vi "Main.vi"() -> ()   [LabVIEW 2019, in "SignalProcessor.lvlib"]
doc: "This template is based off of the Queued Message Handler design pattern and the Queued Message Handler project template that ships with LabVIEW.\n\nThe main difference is that the queue is private to this module and communication between modules is performed via Broadcast and Request events.\n\nRequest events are wrapped in public API methods and are handled in the Event Handling Loop (EHL) of this VI. Any module can register for Broadcast events sent by this module. The EHL generates messages based on user interface actions.\n\nThe Message Handling Loop (MHL) processes messages generated by the EHL, or by other messages. The messages are string values, so new messages can be added easily to the Message Cases case structure in the MHL. Each message cluster can also provide an optional value for Message Data, which is a variant that can be converted to whatever message-specific data is required.\n_____\nBased on Delacor QMH Project Template 4.2.1.64."
uses:
  SignalProcessor.lvlib
  <vilib>/Delacor/Delacor QMH/Libraries/Module Admin_class/Delacor_lib_QMH_Module Admin.lvclass
  Module Data--cluster.ctl
  <vilib>/Delacor/Delacor QMH/Libraries/Message Queue_class/Delacor_lib_QMH_Message Queue.lvclass/Delacor_lib_QMH_Message Queue.ctl
  Stop Argument--cluster.ctl
  <vilib>/Delacor/Delacor QMH/Libraries/Module Admin_class/Delacor_lib_QMH_Module Admin.lvclass/Delacor_lib_QMH_Module Admin.ctl
  ProcessWaveform Argument--cluster.ctl
  <vilib>/Utility/miscctls.llb/LVPointTypeDef.ctl
  <vilib>/Delacor/Delacor QMH/Libraries/Message Queue_class/Delacor_lib_QMH_Enqueue Message (Single).vi
  <vilib>/Delacor/Delacor QMH/Libraries/Module Admin_class/Delacor_lib_QMH_Get External Launch.vi
  <vilib>/Analysis/baseanly.llb/Mean (DBL).vi
  <vilib>/Analysis/5stat.llb/RMS (DBL).vi
  <vilib>/Utility/error.llb/Error Cluster From Error Code.vi
  <vilib>/Waveform/WDTOps.llb/WDT Waveform Duration DBL.vi
  <vilib>/ErrorRing/Error Ring.xnode
  <vilib>/Delacor/Delacor QMH/Libraries/Message Queue_class/Delacor_lib_QMH_Message Queue.lvclass
  <vilib>/Analysis/NI_AALPro.lvlib
  <vilib>/Analysis/NI_AALBase.lvlib
panel:
  in  "Simulate MHL Error":bool
  in  "Simulate EHL Error":bool
  out "error out":errorcluster
  in  "Module Admin":refnum<class "Delacor_lib_QMH_Module Admin.lvclass">
  out "Status":string
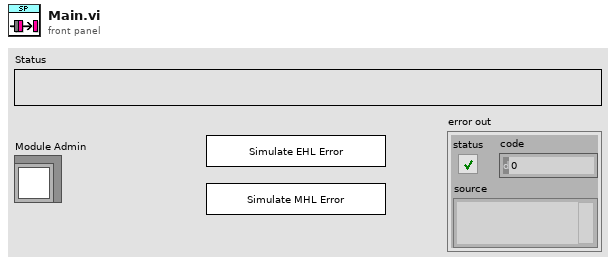
[diagram p1: front panel]
types:
  T1 = typedef "SignalProcessor.lvlib/Request Events--cluster.ctl" = cluster{"Stop Module":refnum<user-event>, "Show Panel":refnum<user-event>, "Hide Panel":refnum<user-event>, "Get Module Execution Status":refnum<user-event>, "Show Diagram":refnum<user-event>, "ProcessWaveform":refnum<user-event>}
  T2 = typedef "SignalProcessor.lvlib/Module Data--cluster.ctl" = cluster{"Status":string}
  T3 = enum32{"invalid lock state", "Not Locked", "Locked (No Password)", "Password-protected"}
  T4 = typedef "SignalProcessor.lvlib/Stop Argument--cluster.ctl" = cluster{"Origin":string, "Exit via Stop Module Req?":bool, "Wait for Module to stop?":bool}
  T5 = typedef "SignalProcessor.lvlib/ProcessWaveform Argument--cluster.ctl" = cluster{"Data":waveform(dbl)}
  T6 = typedef "LVPointTypeDef.ctl" = cluster{"Horizontal":i16, "Vertical":i16}
  T7 = enum32{"Invalid", "Standard", "Closed", "Hidden", "Minimized", "Maximized"}
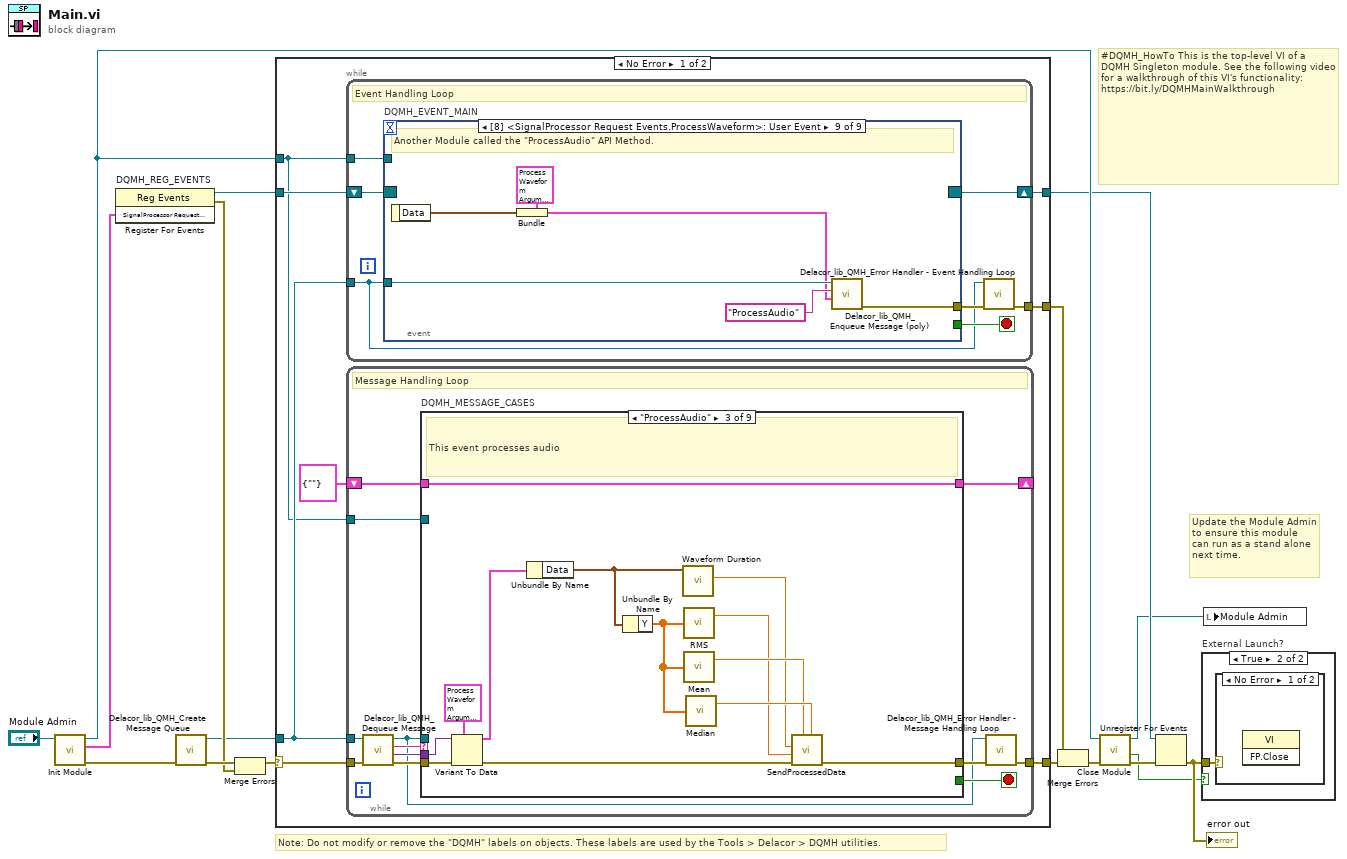
[diagram p0: block diagram]
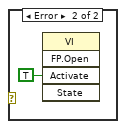
[diagram p3: hidden frame]
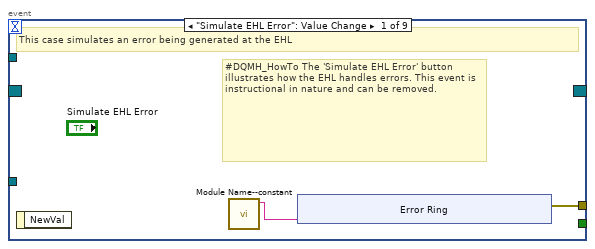
[diagram p4: hidden frame]
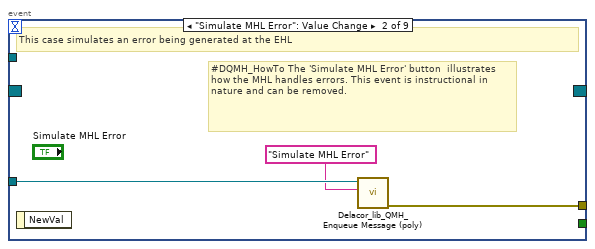
[diagram p5: hidden frame]
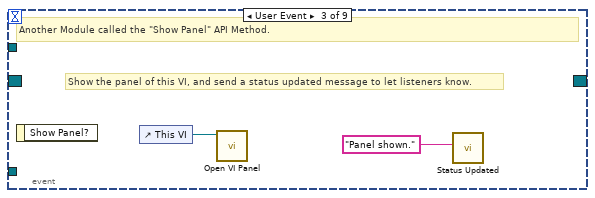
[diagram p6: hidden frame]
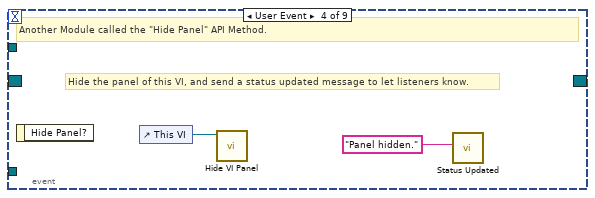
[diagram p7: hidden frame]
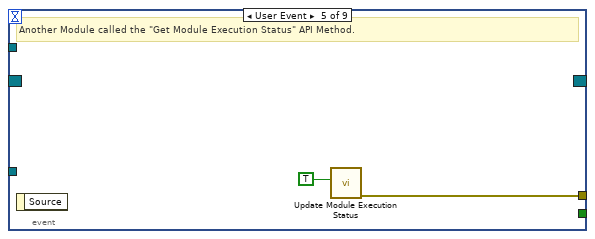
[diagram p8: hidden frame]
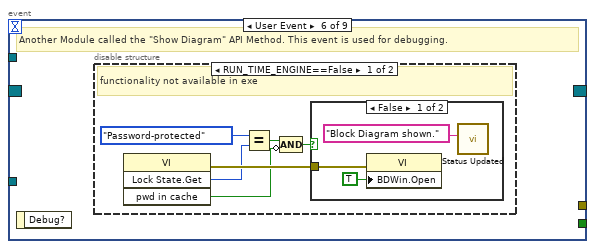
[diagram p9: hidden frame]
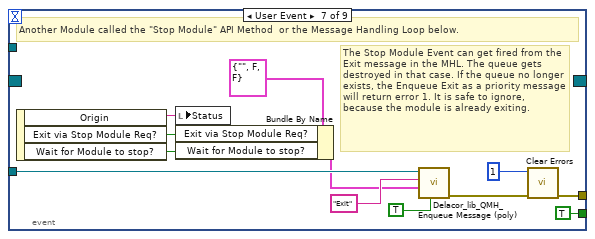
[diagram p12: hidden frame]
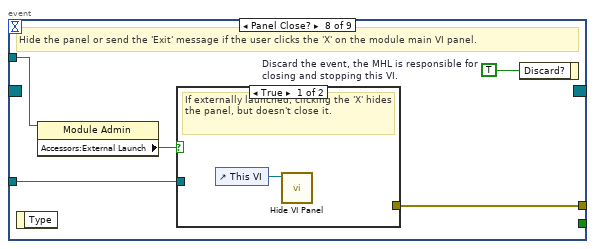
[diagram p13: hidden frame]
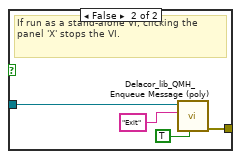
[diagram p14: hidden frame]
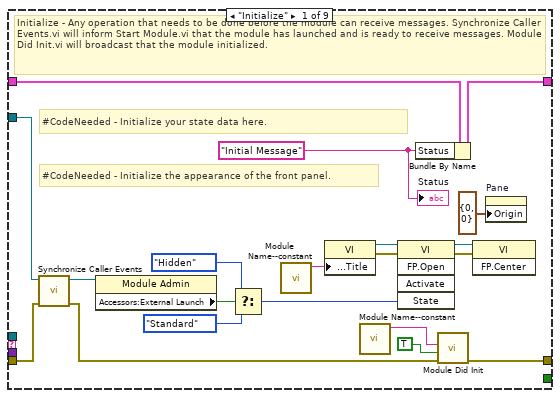
[diagram p15: hidden frame]
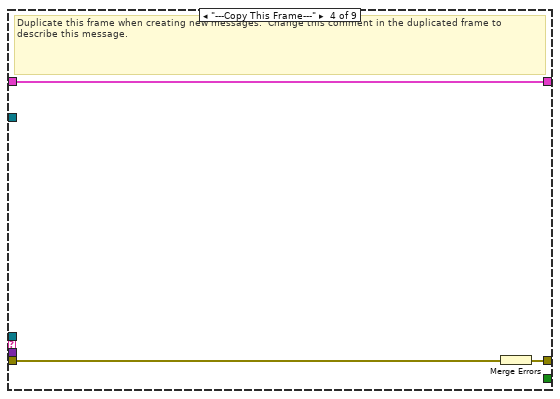
[diagram p17: hidden frame]
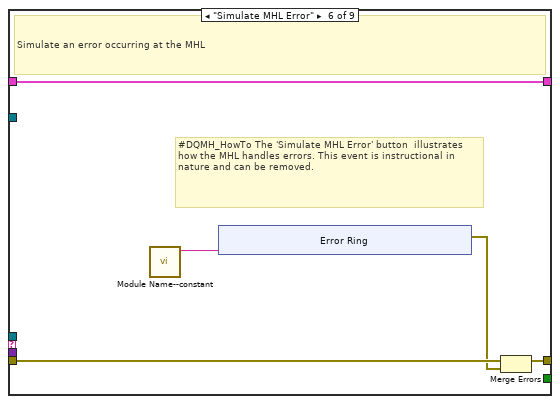
[diagram p19: hidden frame]
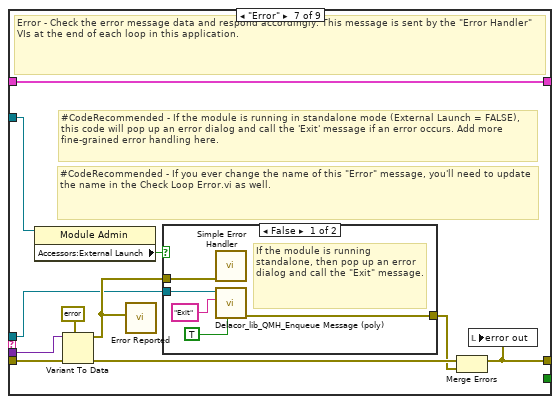
[diagram p20: hidden frame]
diagram:
  # "#DQMH_HowTo This is the top-level VI of a DQMH Singleton module. See the following video for a walkthrough of this VI's functionality: https://bit.ly/DQMHMainWalkthrough"
  # "Note: Do not modify or remove the \"DQMH\" labels on objects. These labels are used by the Tools > Delacor > DQMH utilities."
  # "Update the Module Admin to ensure this module can run as a stand alone next time."
  n1 = call "Init Module.vi"("Singleton Module Admin in"="Module Admin") -> ("error out"=w16:errorcluster, "SignalProcessor Request Events"=w5:T1, "Singleton Module Admin out"=w8:refnum<class "Delacor_lib_QMH_Module Admin.lvclass">)  [unwired: 8 in]
  n2 = register-events "DQMH_REG_EVENTS"(w5) -> (reference out=w6:refnum<event-registration>, error out=w9:errorcluster)  [unwired: 2 in]
  n3 = call <vilib>:"Delacor_lib_QMH_Create Message Queue.vi"("error in (no error)"=w16) -> ("error out"=w11:errorcluster, "Message Queue"=w4:refnum<class "Delacor_lib_QMH_Message Queue.lvclass">)  [unwired: 9 in]
  n4 = Merge Errors(w11, w9) -> (w10:errorcluster)
  n5 = case shown="No Error" w10 {
    selector: w10 -> [w23 w204]
    tunnel: [w25 w204] -> w17
    tunnel: [w22 w201] -> w7
    tunnel: w6 -> [w20 w201]
    tunnel: w4 -> [w19 _]
    tunnel: [w24 _] -> w14
    tunnel: w8 -> [w18 w197]
    frame No Error {
      n6 = while {
        tunnel: w19 -> [w26]
        shift-right: [w29] -> w22
        shift-left: w20 -> [w30]
        tunnel: [w31] -> w24
        tunnel: w18 -> [w27]
        stop <- w28 stop-if-true
        # "Event Handling Loop"
        n7 = event "DQMH_EVENT_MAIN" shown="[8] <SignalProcessor Request Events.ProcessWaveform>: User Event" {
          selector: w30 -> [_ _ _ _ _ _ _ _ _]
          dyn-events: [_ _ _ _ _ _ _ _ _] -> w29
          timeout: _ -> [_ _ _ _ _ _ _ _ _]
          tunnel: [_ _ _ _ _ _ TRUE ("Discard?") _ _] -> w28
          tunnel: w26 -> [_ w43 _ _ _ _ w67 w74 w87]
          tunnel: [w34 w44 _ _ w50 _ w70 w76 w82] -> w32
          tunnel: w27 -> [_ _ _ _ _ _ _ w73 _]
          event "Simulate EHL Error": Value Change {
            # "#DQMH_HowTo The 'Simulate EHL Error' button  illustrates how the EHL handles errors. This event is instructional in nature and can be removed."
            # "This case simulates an error being generated at the EHL"
            n8 = event-data() -> ()  [unwired: 1 in, 1 out]
            n9 = call "Module Name--constant.vi"() -> ("Module Name"=w33:string)  [unwired: 11 in]
            n10 = xnode "Error Ring"("parameter 0"=w33) -> ("error out"=w34:errorcluster)
          }
          event "Simulate MHL Error": Value Change {
            # "#DQMH_HowTo The 'Simulate MHL Error' button  illustrates how the MHL handles errors. This event is instructional in nature and can be removed."
            # "This case simulates an error being generated at the EHL"
            n11 = event-data() -> ()  [unwired: 1 in, 1 out]
            n12 = call-poly <vilib>:"Delacor_lib_QMH_Enqueue Message (poly).vi"("Message"="Simulate MHL Error", "Message Queue in"=w43) -> ("error out"=w44:errorcluster)  [unwired: 8 in, 1 out]
          }
          event User Event {
            # "Show the panel of this VI, and send a status updated message to let listeners know."
            # "Another Module called the \"Show Panel\" API Method."
            n13 = event-data() -> ()  [unwired: 1 in, 1 out]
            n14 = control-ref of="This VI"() -> (w46:refnum<vi>)
            n15 = call "Open VI Panel.vi"("VI"=w46) -> ()  [unwired: 10 in, 1 out]
            n16 = call "Status Updated.vi"("Status"="Panel shown." ("format string")) -> ()  [unwired: 10 in, 1 out]
          }
          event User Event {
            # "Hide the panel of this VI, and send a status updated message to let listeners know."
            # "Another Module called the \"Hide Panel\" API Method."
            n17 = event-data() -> ()  [unwired: 1 in, 1 out]
            n18 = control-ref of="This VI"() -> (w48:refnum<vi>)
            n19 = call "Hide VI Panel.vi"("VI"=w48) -> ()  [unwired: 10 in, 1 out]
            n20 = call "Status Updated.vi"("Status"="Panel hidden." ("format string")) -> ()  [unwired: 10 in, 1 out]
          }
          event User Event {
            # "Another Module called the \"Get Module Execution Status\" API Method."
            n21 = event-data() -> ()  [unwired: 1 in, 1 out]
            n22 = call "Update Module Execution Status.vi"("Running?"=TRUE) -> ("error out"=w50:errorcluster)  [unwired: 10 in]
          }
          event User Event {
            # "Another Module called the \"Show Diagram\" API Method. This event is used for debugging."
            n23 = event-data() -> ()  [unwired: 1 in, 1 out]
            n24 = disable-structure shown="RUN_TIME_ENGINE==False" {
              frame condition #0 (active) {
                # "functionality not available in exe"
                n25 = invoke class="VI" method="Lock State.Get"() -> (error out=w56:errorcluster, "Get Lock State"=w55:T3, "pwd in cache"=w52:bool)  [unwired: 4 in, 1 out]
                n26 = Equal?(x=T3."Password-protected", y=w55) -> (x = y?=w53:bool)
                n27 = Compound Arithmetic op=AND(w53, invert w52) -> (w51:bool)
                n28 = case shown="False" w51 {
                  tunnel: w56 -> [w59 _]
                  frame False {
                    n29 = property class="VI"(error in=w59, "BDWin.Open"=TRUE ("Block Diagram Window:Open")) -> ()  [unwired: 1 in, 2 out]
                    n30 = call "Status Updated.vi"("Status"="Block Diagram shown." ("format string")) -> ()  [unwired: 10 in, 1 out]
                  }
                  frame True {
                    # "Password-protected VI, and the password is not in the cache. Do not show the diagram."
                  }
                }
              }
              frame condition #1 {
              }
            }
          }
          event User Event {
            # "The Stop Module Event can get fired from the Exit message in the MHL. The queue gets destroyed in that case. If the queue no longer exists, the Enqueue Exit as a priority message will return error 1. It is safe to ignore, because the module is already exiting."
            # "Another Module called the \"Stop Module\" API Method  or the Message Handling Loop below."
            n31 = event-data() -> ("Origin"=w66:string, "Exit via Stop Module Req?"=w62:bool, "Wait for Module to stop?"=w61:bool)  [unwired: 1 in]
            n32 = local write "Status"(w66) -> ()
            n33 = Bundle By Name(cluster=T4 {"Origin"="", "Exit via Stop Module Req?"=FALSE, "Wait for Module to stop?"=FALSE} ("Stop Argument"), "Exit via Stop Module Req?"=w62, "Wait for Module to stop?"=w61) -> (w60:T4)
            n34 = call-poly <vilib>:"Delacor_lib_QMH_Enqueue Message (poly).vi"("Priority Message? (F)"=TRUE, "Message Data"=w60, "Message"="Exit", "Message Queue in"=w67) -> ("error out"=w71:errorcluster)  [unwired: 6 in, 1 out]
            n35 = call <vilib>:"Clear Errors.vi"("error in (no error)"=w71, "specific error code to clear (0: all)"=1) -> ("error out"=w70:errorcluster)  [unwired: 4 in, 1 out]
          }
          event Panel Close? {
            w75 = TRUE  # Discard the event, the MHL is responsible for closing and stopping this VI.
            # "Hide the panel or send the 'Exit' message if the user clicks the 'X' on the module main VI panel."
            n36 = event-data() -> ()  [unwired: 1 in, 1 out]
            n37 = property class="Module Admin"(reference=w73) -> ("Accessors:External Launch"=w72:bool)  [unwired: 1 in, 2 out]
            n38 = case shown="True" w72 {
              tunnel: w74 -> [_ w80]
              tunnel: [_ w81] -> w76
              frame True {
                # "If externally launched, clicking the 'X' hides the panel, but doesn't close it."
                n39 = control-ref of="This VI"() -> (w77:refnum<vi>)
                n40 = call "Hide VI Panel.vi"("VI"=w77) -> ()  [unwired: 10 in, 1 out]
              }
              frame False {
                # "If run as a stand-alone VI, clicking the panel 'X' stops the VI."
                n41 = call-poly <vilib>:"Delacor_lib_QMH_Enqueue Message (poly).vi"("Priority Message? (F)"=TRUE, "Message"="Exit", "Message Queue in"=w80) -> ("error out"=w81:errorcluster)  [unwired: 7 in, 1 out]
              }
            }
            n42 = event-data("Discard?"=w75) -> ()  [unwired: 1 in, 1 out]
          }
          event User Event {
            # "Another Module called the \"ProcessAudio\" API Method."
            n43 = event-data() -> ("Data"=w83:waveform(dbl))  [unwired: 1 in]
            n44 = Bundle(cluster=T5 {"Data"={"t0"=timestamp(0 s since 1904-01-01), "dt"=1.0, "Y"=[]}} ("ProcessAudio Argument"), "Data"=w83) -> (w84:T5)
            n45 = call-poly <vilib>:"Delacor_lib_QMH_Enqueue Message (poly).vi"("Message Data"=w84, "Message"="ProcessAudio", "Message Queue in"=w87) -> ("error out"=w82:errorcluster)  [unwired: 7 in, 1 out]
          }
        }
        n46 = call-dynamic "Delacor_lib_QMH_Error Handler - Event Handling Loop.vi"("error in (no error)"=w32, "Message Queue in"=w26) -> ("dup error in"=w31:errorcluster)  [unwired: 8 in, 1 out]
      }
      n47 = while {
        tunnel: w19 -> [w90]
        shift-right: [w94] -> _
        shift-left: T2 {"Status"=""} ("Data Cluster") -> [w95]
        tunnel: w23 -> [w98]
        tunnel: [w96] -> w25
        tunnel: w18 -> [w88]
        stop <- w93 stop-if-true
        # "Message Handling Loop"
        n48 = call-dynamic "Delacor_lib_QMH_Dequeue Message.vi"("error in (no error)"=w98, "Message Queue in"=w90) -> ("error out"=w97:errorcluster, "Message Data"=w91:variant, "Message"=w92:string, "Message Queue out"=w89:refnum<class "Delacor_lib_QMH_Message Queue.lvclass">)  [unwired: 6 in]
        n49 = case "DQMH_MESSAGE_CASES" shown="\"ProcessAudio\"" w92 {
          selector: w92 -> [_ _ _ _ _ _ _ _ w184]
          tunnel: w89 -> [_ _ _ _ _ _ w154 w176 _]
          tunnel: w97 -> [w117 w121 w134 w137 w139 w144 w161 w182 w186]
          tunnel: [w115 w121 w126 w136 w139 w143 w157 w179 w187] -> w99
          tunnel: w95 -> [w106 w120 w133 w135 w138 w141 w156 w175 w185]
          tunnel: [w105 w120 w133 w135 w138 w141 w156 w175 w185] -> w94
          tunnel: [_ _ _ _ _ _ _ w174 _] -> w93
          tunnel: w91 -> [_ _ w132 _ _ _ w155 w173 _]
          tunnel: w88 -> [w107 _ _ _ _ _ w153 w168 _]
          frame "Initialize" {
            w100 = "Initial Message" ("Initial Message")
            # "#CodeNeeded - Initialize the appearance of the front panel."
            # "#CodeNeeded - Initialize your state data here."
            # "Initialize - Any operation that needs to be done before the module can receive messages. Synchronize Caller Events.vi will inform Start Module.vi that the module has launched and is ready to receive messages. Module Did Init.vi will broadcast that the module initialized."
            n50 = call "Synchronize Caller Events.vi"("error in (no error)"=w117, "Singleton Module Admin in"=w107) -> ("error out"=w116:errorcluster, "Singleton Module Admin out"=w102:refnum<class "Delacor_lib_QMH_Module Admin.lvclass">)  [unwired: 8 in]
            n51 = property class="Module Admin"(reference=w102) -> ("Accessors:External Launch"=w111:bool)  [unwired: 1 in, 2 out]
            n52 = Select(t=T7."Hidden" ("State"), s=w111, f=T7."Standard" ("State")) -> (s? t:f=w108:T7)
            n53 = call "Module Name--constant.vi"() -> ("Module Name"=w114:string)  [unwired: 11 in]
            n54 = property class="VI"("Front Panel.Title"=w114) -> (reference out=w113:refnum<vi>, error out=w119:errorcluster)  [unwired: 2 in]
            n55 = call "Module Name--constant.vi"() -> ("Module Name"=w103:string)  [unwired: 11 in]
            n56 = invoke class="VI" method="FP.Open"(reference=w113, error in=w119, "State"=w108) -> (reference out=w112:refnum<vi>, error out=w118:errorcluster)  [unwired: 2 in, 3 out]
            n57 = Bundle By Name(cluster=w106, "Status"=w100) -> (w105:T2)
            n58 = call "Module Did Init.vi"("error in (no error)"=w116, "Initialized?"=TRUE, "Origin"=w103) -> ("error out"=w115:errorcluster)  [unwired: 8 in]
            n59 = invoke class="VI" method="FP.Center"(reference=w112, error in=w118) -> ()  [unwired: 1 in, 3 out]
            n60 = property on="Pane" class="Pane"("Origin"=T6 {"Horizontal"=0, "Vertical"=0}) -> ()  [unwired: 2 in, 2 out]
            "Status" <- w100
          }
          frame "--- Module Specific ---" {
            # "Separator -- The following cases handle messages specific to this Module."
          }
          frame "ProcessAudio" {
            # "This event processes audio"
            n61 = Variant To Data(error in=w134, type=T5 {"Data"={"t0"=timestamp(0 s since 1904-01-01), "dt"=1.0, "Y"=[]}} ("ProcessAudio Argument"), Variant=w132) -> (data=w130:T5, error out=w127:errorcluster)
            n62 = Unbundle By Name(w130) -> ("Data"=w129:waveform(dbl))
            n63 = Unbundle By Name(w129) -> ("Y"=w128:dbl[])
            n64 = call-poly <vilib>:"Waveform Duration.vi"("waveform in"=w129) -> ("duration"=w123:dbl)  [unwired: 8 in, 2 out]
            n65 = call-poly <vilib>:"RMS.vi"("X"=w128) -> ("rms value"=w122:dbl)  [unwired: 1 out]
            n66 = call-poly <vilib>:"Mean.vi"("X"=w128) -> ("mean"=w124:dbl)  [unwired: 1 out]
            n67 = call <vilib>:"Median.vi"("X"=w128) -> ("median"=w125:dbl)  [unwired: 1 out]
            n68 = call "SendProcessedData.vi"("Median"=w125, "Mean"=w124, "error in (no error)"=w127, "RMS"=w122, "Duration"=w123) -> ("error out"=w126:errorcluster)  [unwired: 6 in]
          }
          frame "---Copy This Frame---" {
            # "Duplicate this frame when creating new messages.  Change this comment in the duplicated frame to describe this message."
            n69 = Merge Errors(w137) -> (w136:errorcluster)
          }
          frame "--- Exit and Error Handling---" {
            # "Separator - The following cases handle errors and exit messages."
          }
          frame "Simulate MHL Error" {
            # "#DQMH_HowTo The 'Simulate MHL Error' button  illustrates how the MHL handles errors. This event is instructional in nature and can be removed."
            # "Simulate an error occurring at the MHL"
            n70 = call "Module Name--constant.vi"() -> ("Module Name"=w140:string)  [unwired: 11 in]
            n71 = xnode "Error Ring"("parameter 0"=w140) -> ("error out"=w142:errorcluster)
            n72 = Merge Errors(w144, w142) -> (w143:errorcluster)
          }
          frame "Error" {
            # "#CodeRecommended - If you ever change the name of this \"Error\" message, you'll need to update the name in the Check Loop Error.vi as well."
            # "#CodeRecommended - If the module is running in standalone mode (External Launch = FALSE), this code will pop up an error dialog and call the 'Exit' message if an error occurs. Add more fine-grained error handling here."
            # "Error - Check the error message data and respond accordingly. This message is sent by the \"Error Handler\" VIs at the end of each loop in this application."
            n73 = property class="Module Admin"(reference=w153) -> ("Accessors:External Launch"=w152:bool)  [unwired: 1 in, 2 out]
            n74 = Variant To Data(error in=w161, type=errorcluster {"status"=FALSE, "code"=0, "source"=""} ("error constant"), Variant=w155) -> (data=w162:errorcluster, error out=w159:errorcluster)
            n75 = call "Error Reported.vi"("Error"=w162) -> ()  [unwired: 10 in, 1 out]
            n76 = case shown="False" w152 {
              tunnel: [w167 _] -> w158
              tunnel: w154 -> [w165 _]
              tunnel: w162 -> [w166 _]
              frame False {
                # "If the module is running standalone, then pop up an error dialog and call the \"Exit\" message."
                n77 = call <vilib>:"Simple Error Handler.vi"("error in (no error)"=w166) -> ()  [unwired: 4 in, 5 out]
                n78 = call-poly <vilib>:"Delacor_lib_QMH_Enqueue Message (poly).vi"("Priority Message? (F)"=TRUE, "Message"="Exit", "Message Queue in"=w165) -> ("error out"=w167:errorcluster)  [unwired: 7 in, 1 out]
              }
              frame True {
                # "If the module was launched externally, calling the Error Reported broadcast VI is the only action performed by the \"Error\" message. The module's caller can then process the error appropriately."
              }
            }
            n79 = Merge Errors(w159, w158) -> (w157:errorcluster)
            n80 = local write "error out"(w157) -> ()
          }
          frame "Exit" {
            w172 = 91  # 91: not all Exit messages will have an argument
            w174 = TRUE  # Stop the VI
            # "Release the message queue reference"
            # "#CodeNeeded - Add any required cleanup code here"
            # "Exit - Exit the application."
            n81 = Variant To Data(error in=w182, type=T4 {"Origin"="", "Exit via Stop Module Req?"=FALSE, "Wait for Module to stop?"=FALSE} ("Stop Argument"), Variant=w173) -> (data=w170:T4, error out=w178:errorcluster)
            n82 = call <vilib>:"Clear Errors.vi"("error in (no error)"=w178, "specific error code to clear (0: all)"=w172) -> ("error out"=w181:errorcluster)  [unwired: 4 in, 1 out]
            n83 = control-ref of="This VI"() -> (w169:refnum<vi>)
            n84 = call-dynamic "Delacor_lib_QMH_Release Message Queue.vi"("error in (no error)"=w181, "Message Queue"=w176) -> ("error out"=w180:errorcluster)  [unwired: 9 in]
            n85 = call "Handle Exit.vi"("Stop Argument"=w170, "Admin in"=w168, "VI reference"=w169) -> ("error out"=w177:errorcluster)  [unwired: 7 in, 1 out]
            n86 = Merge Errors(w180, w177) -> (w179:errorcluster)
          }
          frame Default {
            # "'Default' case only runs if there is a message that isn't defined in any of the other cases.  Output a programming error."
            n87 = call "Module Name--constant.vi"() -> ("Module Name"=w183:string)  [unwired: 11 in]
            n88 = xnode "Error Ring"("parameter 0"=w184, "parameter 1"=w183) -> ("error out"=w188:errorcluster)
            n89 = Merge Errors(w186, w188) -> (w187:errorcluster)
          }
        }
        n90 = call-dynamic "Delacor_lib_QMH_Error Handler - Message Handling Loop.vi"("error in (no error)"=w99, "Message Queue in"=w89) -> ("dup error in"=w96:errorcluster)  [unwired: 8 in, 1 out]
      }
    }
    frame Error {
      # "Synchronize Caller Events.vi will inform Start Module.vi that the module has launched and will let the code calling Start Module.vi register for broadcasts and would permit the caller receive the broadcast that an error occurred at launch time."
      n91 = call "Synchronize Caller Events.vi"("Singleton Module Admin in"=w197) -> ("error out"=w202:errorcluster)  [unwired: 9 in, 1 out]
      n92 = call "Module Name--constant.vi"() -> ("Module Name"=w200:string)  [unwired: 11 in]
      n93 = Format Into String(format string="An error occurred during initialization. %s is no longer running.", w200) -> (resulting string=w198:string)  [unwired: 2 in, 1 out]
      n94 = Merge Errors(w204, w202) -> (w203:errorcluster)
      n95 = call "Error Reported.vi"("Additional Information"=w198, "Error"=w203) -> ()  [unwired: 9 in, 1 out]
    }
  }
  n96 = Merge Errors(w14, w17) -> (w13:errorcluster)
  n97 = call "Close Module.vi"("error in (no error)"=w13, "Module Admin in"=w8) -> ("error out"=w15:errorcluster, "External Launch"=w1:bool, "Module Admin out"=w2:refnum<class "Delacor_lib_QMH_Module Admin.lvclass">)  [unwired: 7 in]
  n98 = Unregister For Events(event registration refnum=w7, error in=w15) -> (error out=w12:errorcluster)
  "error out" <- w12
  n99 = case "External Launch?" shown="True" w1 {
    tunnel: w12 -> [_ w205]
    frame False {
    }
    frame True {
      n100 = case shown="No Error" w205 {
        frame No Error {
          n101 = invoke class="VI" method="FP.Close"() -> ()  [unwired: 3 in, 3 out]
        }
        frame Error {
          n102 = invoke class="VI" method="FP.Open"("Activate"=TRUE ("Activate?")) -> ()  [unwired: 4 in, 5 out]
        }
      }
    }
  }
  n103 = local write "Module Admin"(w2) -> ()
